vi "FTW-Endpoint-Multipart-Ask.vi"(0 "FTW ØMQ Endpoint":refnum<class "FTW-Endpoint-ZMQ.lvclass">, 5 "Multipart Message":string[](array[string]), 7 "Read Timeout":i32=100 format="%dmsec", 9 "Write Timeout":i32 format="%dmsec", 11 "error in":errorcluster) -> (4 "FTW ØMQ Endpoint out":refnum<class "FTW-Endpoint-ZMQ.lvclass">, 6 "Reply":string[](array[string]), 8 "Read Timed out?":bool, 10 "Write Timed out?":bool, 15 "error out":errorcluster)   [LabVIEW 2012, in "FTW-Actor.lvlib" / "FTW-Endpoint-ZMQ.lvclass"]
uses:
  FTW-Endpoint-ZMQ.lvclass
  FTW-Endpoint-ZMQ.lvclass/FTW-Endpoint-ZMQ.ctl
  FTW-ZMQ-LibraryFilepath.vi
  FTW-ZMQ-LibraryReturnValue.vi
panel:
  # "Inputs"
  # "Outputs"
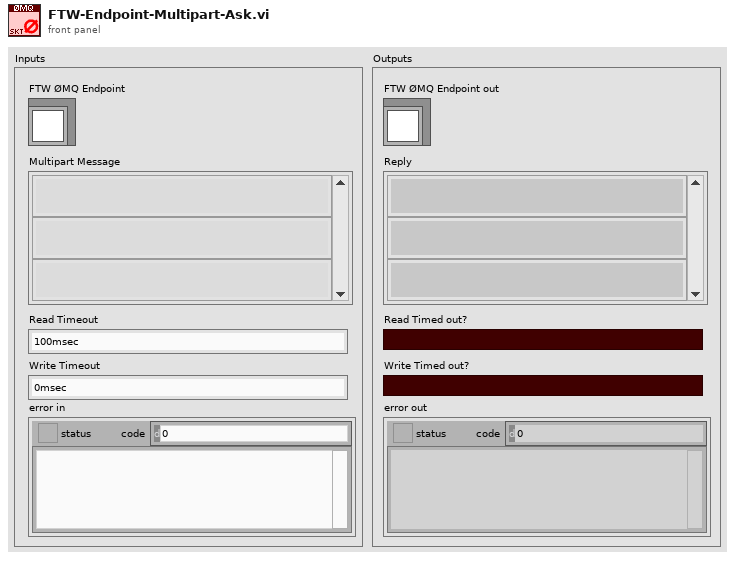
[diagram p1: front panel]
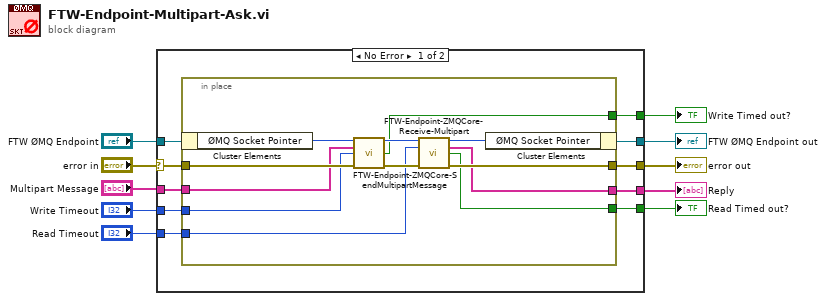
[diagram p0: block diagram]
diagram:
  n1 = case shown="No Error" "error in" {
    selector: "error in" -> [w16 w33]
    tunnel: "FTW ØMQ Endpoint" -> [w20 w34]
    tunnel: "Multipart Message" -> [w19 _]
    tunnel: [w18 w33] -> w5
    tunnel: [w17 w34] -> w6
    tunnel: "Read Timeout" -> [w15 _]
    tunnel: [w14 _] -> w4
    tunnel: [w13 _] -> w3
    tunnel: "Write Timeout" -> [w12 _]
    tunnel: [w11 _] -> w1
    frame No Error {
      n2 = in-place {
        in-place-border: w19 -> [w30]
        in-place-border: w16 -> [w32]
        in-place-border: [w25] -> w18
        in-place-border: w15 -> [w26]
        in-place-border: [w24] -> w14
        in-place-border: [w23] -> w13
        in-place-border: w12 -> [w22]
        in-place-border: [w21] -> w11
        n3 = in-place-cluster #1(w20) -> ("ØMQ Socket Pointer"=w31:u64)
        n4 = call "FTW-Endpoint-ZMQCore-SendMultipartMessage.vi"("ØMQ Socket Pointer"=w31, "Multipart Message"=w30, "Write Timeout"=w22, "error in"=w32) -> ("ØMQ Socket Pointer out"=w29:u64, "Write Timed out?"=w21:bool, "error out"=w27:errorcluster)  [unwired: 9 in]
        n5 = call "FTW-Endpoint-ZMQCore-Receive-Multipart.vi"("ØMQ Socket Pointer"=w29, "Timeout"=w26, "error in"=w27) -> ("ØMQ Socket Pointer out"=w28:u64, "Multipart Message"=w24:string[], "Timed out?"=w23:bool, "error out"=w25:errorcluster)  [unwired: 9 in]
        n6 = in-place-cluster #1("ØMQ Socket Pointer"=w28) -> (w17:refnum<class "FTW-Endpoint-ZMQ.lvclass">)
      }
    }
    frame Error {
    }
  }
  "error out" <- w5
  "FTW ØMQ Endpoint out" <- w6
  "Read Timed out?" <- w3
  "Reply" <- w4
  "Write Timed out?" <- w1
